vi "Build_tdms_ch_name.vi"(11 "Frame_nb":i32) -> (3 "Channel_name":string[](array[string]))   [LabVIEW 2019]
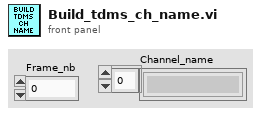
[diagram p1: front panel]
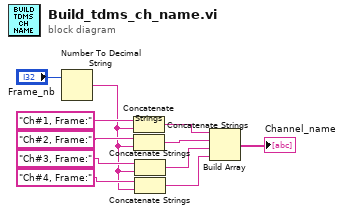
[diagram p0: block diagram]
diagram:
  n1 = Number To Decimal String(number="Frame_nb") -> (decimal integer string=w3:string)  [unwired: 1 in]
  n2 = Concatenate Strings("Ch#1, Frame:" ("group name in (Untitled)"), w3) -> (w9:string)
  n3 = Concatenate Strings("Ch#2, Frame:" ("group name in (Untitled)"), w3) -> (w11:string)
  n4 = Concatenate Strings("Ch#3, Frame:" ("group name in (Untitled)"), w3) -> (w2:string)
  n5 = Concatenate Strings("Ch#4, Frame:" ("group name in (Untitled)"), w3) -> (w1:string)
  n6 = Build Array(w9, w11, w2, w1) -> (→"Channel_name":string[])
